vi "setX.vi"(8 "error in (no error)":errorcluster, 10 "x":i32, 11 "fwCircle in":refnum<class "fwCircle.lvclass">) -> (0 "error out":errorcluster, 3 "fwCircle out":refnum<class "fwCircle.lvclass">)   [LabVIEW 2016, in "fwCircle.lvclass"]
uses:
  fwCircle.lvclass
  fwCircle.lvclass/fwCircle.ctl
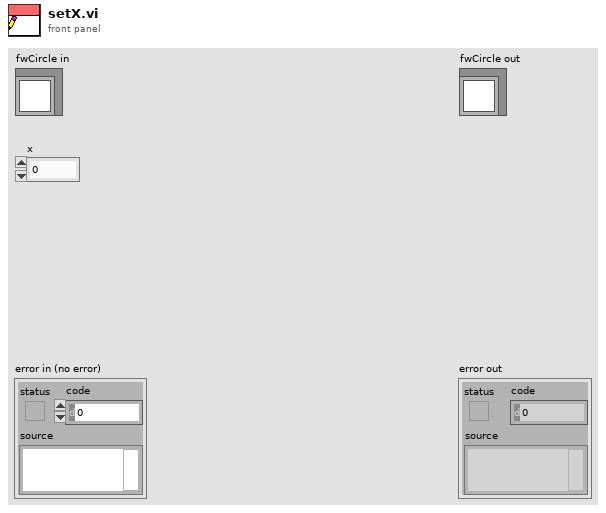
[diagram p1: front panel]
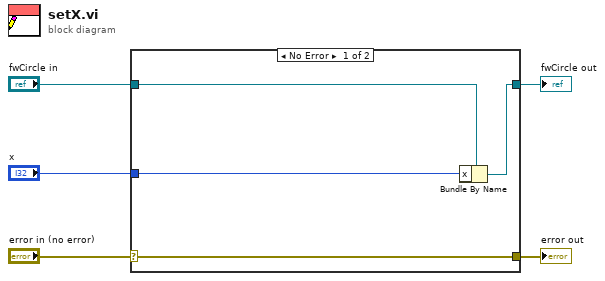
[diagram p0: block diagram]
diagram:
  n1 = case shown="No Error" "error in (no error)" {
    selector: "error in (no error)" -> [w9 w10]
    tunnel: [w9 w10] -> w4
    tunnel: [w7 w11] -> w2
    tunnel: "fwCircle in" -> [w8 w11]
    tunnel: "x" -> [w6 _]
    frame No Error {
      n2 = Bundle By Name(cluster=w8, "x"=w6) -> (w7:refnum<class "fwCircle.lvclass">)
    }
    frame Error {
    }
  }
  "error out" <- w4
  "fwCircle out" <- w2
